vi "Auto-Fill.vi"() -> ()   [LabVIEW 2011]
uses:
  SubVI/Auto-Fill Cases.ctl
  SubVI/Valve_Pump.ctl
  SubVI/Pumps_Valves_Dependencies_Global.vi
panel:
  out "Output Height cm":dbl
  out "Litre":dbl
  in  "Emergency Stop":bool
  out "Litres":dbl(slide) scale=0.0..14400.0
  out "Tank C":dbl(slide) scale=0.0..100.0
  out "Tank B":dbl(slide) scale=0.0..100.0
  out "Tank D":dbl(slide) scale=0.0..100.0
  out "Tank A":dbl(slide) scale=0.0..100.0
  in  "Density (kg/m3)":dbl[](array[numeric])=[0.0, 0.0, 0.0, 0.0, 0.0, 0.0]
  in  "Height (cm)":dbl[](array[numeric])=[0.0, 0.0, 0.0, 0.0, 0.0, 0.0]
  in  "Auto-Fill":T1
  in  "Start Process":bool
  # "Enter density required in \nascending order"
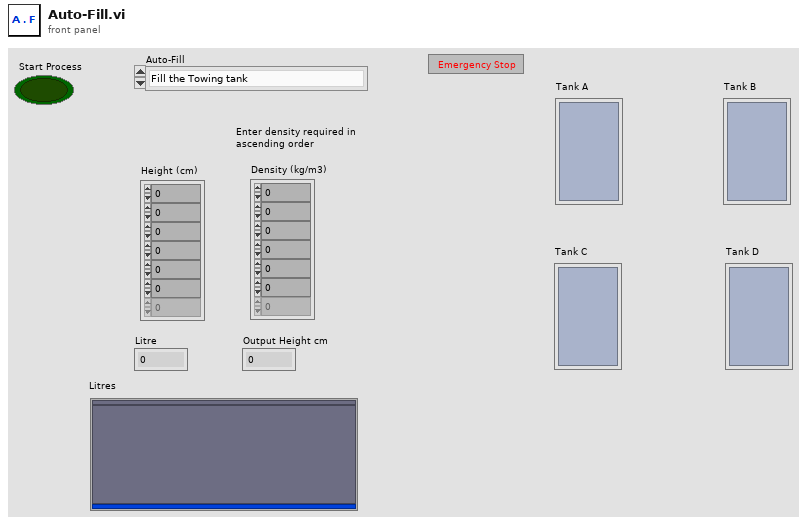
[diagram p1: front panel]
types:
  T1 = typedef "Auto-Fill Cases.ctl" = enum16{"Fill the Towing tank", "Fill Tank A from the Salt saturator tank", "Fill Tank B from the Salt Saturator tank", "Fill Tank C from the water mains", "Fill Tank D from the water mains", "Fill tank B from tank A", "Fill tank C from tank D"}
  T2 = typedef "Valve_Pump.ctl" = enum16{"Main Rack Power", "Pump Power", "Valve Power", "V4", "V5", "V6", "V7", "V8", "V9", "V10", "V11", "V12", "V13", "V14", "V15", "V18", "V19", "V20", "V21", "V22", "V23", "V24", "V25", "V26", "V27", "V28", "V29", "V30", "V31", "V32", "V33", "V34", "Pump A", "Pump B", "Pump C", "Pump D"}
  T3 = cluster{"Tanks[0]":dbl, "Tanks[1]":dbl, "Tanks[2]":dbl, "Tanks[3]":dbl, "Tanks[4]":dbl}
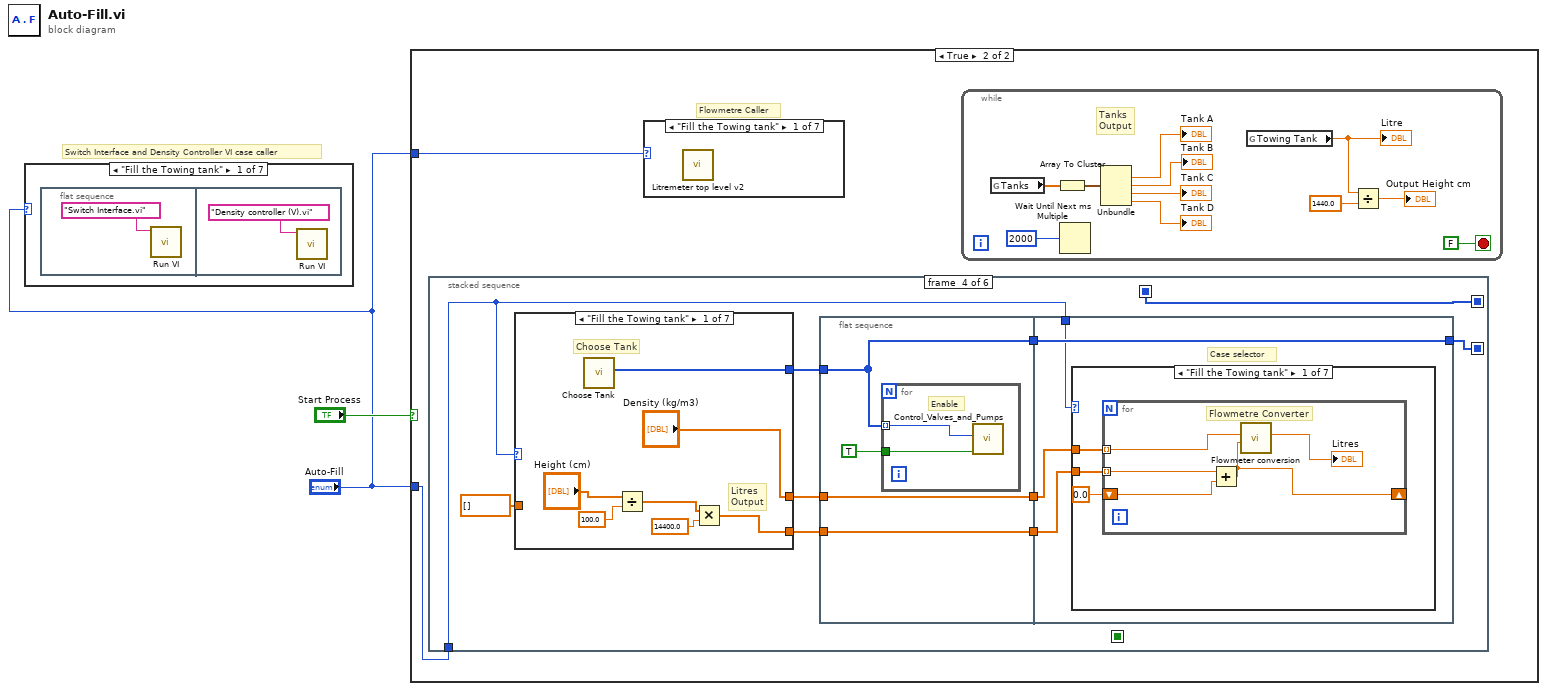
[diagram p0: block diagram]
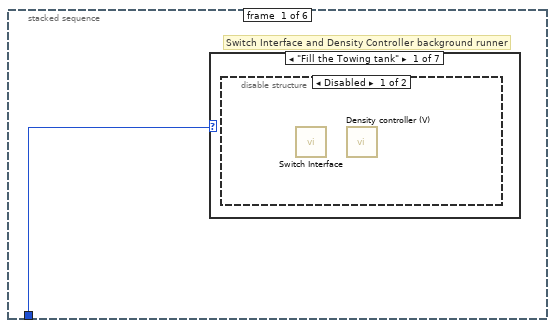
[diagram p15: hidden frame]
diagram:
  # "Switch Interface and Density Controller VI case caller"
  n1 = case shown="\"Fill the Towing tank\"" "Auto-Fill" {
    frame "Fill the Towing tank" {
      n2 = flat-sequence {
        frame #0 {
          n3 = call "Run VI.vi"("VI name"="Switch Interface.vi") -> ()  [unwired: 11 in]
        }
        frame #1 {
          n4 = call "Run VI.vi"("VI name"="Density controller (V).vi") -> ()  [unwired: 11 in]
        }
      }
    }
    frame "Fill Tank A from the Salt saturator tank" {
    }
    frame "Fill Tank B from the Salt Saturator tank" {
    }
    frame "Fill Tank C from the water mains" {
    }
    frame "Fill Tank D from the water mains" {
    }
    frame "Fill tank B from tank A" {
    }
    frame "Fill tank C from tank D" {
    }
  }
  n5 = case shown="True" "Start Process" {
    tunnel: "Auto-Fill" -> [_ w6]
    tunnel: "Auto-Fill" -> [_ w5]
    frame False {
    }
    frame True {
      # "Flowmetre Caller"
      n6 = stacked-sequence {
        seq-local: [_ _ w24 _ _ _] -> [_ _ _ w37 _ _]
        seq-local: [_ _ _ w34 _ _] -> [_ _ _ _ w144 _]
        seq-local: [_ _ _ w37 _ _] -> [_ _ _ _ w143 _]
        seq-local: [_ _ _ _ w140 _] -> [_ _ _ _ _ w148]
        tunnel: w6 -> [w18 _ _ w28 _ _]
        frame #0 {
          # "Switch Interface and Density Controller background runner"
          n7 = case shown="\"Fill the Towing tank\"" w18 {
            frame "Fill the Towing tank" {
              n8 = disable-structure shown="Disabled" {
                frame Disabled {
                  n9 = call "Switch Interface.vi"() -> ()  [unwired: 12 in]
                  n10 = call "Density controller (V).vi"() -> ()  [unwired: 12 in]
                }
                frame Enabled {
                }
              }
            }
            frame "Fill Tank A from the Salt saturator tank" {
            }
            frame "Fill Tank B from the Salt Saturator tank" {
            }
            frame "Fill Tank C from the water mains" {
            }
            frame "Fill Tank D from the water mains" {
            }
            frame "Fill tank B from tank A" {
            }
            frame "Fill tank C from tank D" {
            }
          }
        }
        frame #1 {
          # "Sequence delay time to allow Switch Interface VI to initialize"
          n11 = Wait (ms)(milliseconds to wait=u32 50000 ("millisecond multiple")) -> ()  [unwired: 1 out]
        }
        frame #2 {
          # "Identifier array\nbuild-up"
          n12 = Build Array(Valve_Pump."Main Rack Power" ("Device"), Valve_Pump."Pump Power" ("Device"), Valve_Pump."Valve Power" ("Device")) -> (w24:T2[])
          n13 = for {
            tunnel: TRUE -> [w26]
            tunnel: w24 -> [w27] mode=indexing
            # "Time delay"
            n14 = call "Control_Valves_and_Pumps.vi"("Set state:"=w26, "Device"=w27) -> ()  [unwired: 10 in]
            n15 = Wait Until Next ms Multiple(millisecond multiple=3000) -> ()  [unwired: 1 out]
          }
        }
        frame #3 {
          n16 = case shown="\"Fill the Towing tank\"" w28 {
            tunnel: [w110 w112 w117 w122 w125 w129 w135] -> w35
            tunnel: [w104 w111 w116 w121 w124 w127 w133] -> w29
            tunnel: ["Density (kg/m3)" w111 w116 w121 w124 w127 w133] -> w32
            tunnel: dbl[] [] ("Density (kg/m3)") -> [_ w111 w116 w121 w124 w127 w133]
            frame "Fill the Towing tank" {
              # "Choose Tank"
              # "Litres\nOutput"
              n17 = call "Choose Tank.vi"() -> ("Device"=w110:T2[])  [unwired: 9 in]
              n18 = Divide(x="Height (cm)", y=100.0) -> (x/y=w106:dbl[])
              n19 = Multiply(x=w106, y=14400.0) -> (x*y=w104:dbl[])
            }
            frame "Fill Tank A from the Salt saturator tank" {
              n20 = Build Array(Valve_Pump."V29" ("Device"), Valve_Pump."V27" ("Device"), Valve_Pump."Pump A" ("Device")) -> (w112:T2[])
            }
            frame "Fill Tank B from the Salt Saturator tank" {
              n21 = Build Array(Valve_Pump."V29" ("Device"), Valve_Pump."V23" ("Device"), Valve_Pump."Pump A" ("Device")) -> (w117:T2[])
            }
            frame "Fill Tank C from the water mains" {
              # "Identifier array\nbuild-up"
              n22 = Build Array(Valve_Pump."V8" ("Device")) -> (w122:T2[])
            }
            frame "Fill Tank D from the water mains" {
              # "Identifier array\nbuild-up"
              n23 = Build Array(Valve_Pump."V10" ("Device")) -> (w125:T2[])
            }
            frame "Fill tank B from tank A" {
              # "Identifier array\nbuild-up"
              n24 = Build Array(Valve_Pump."V4" ("Device"), Valve_Pump."V20" ("Device"), Valve_Pump."V22" ("Device"), Valve_Pump."Pump B" ("Device")) -> (w129:T2[])
            }
            frame "Fill tank C from tank D" {
              # "Identifier array\nbuild-up"
              n25 = Build Array(Valve_Pump."V9" ("Device"), Valve_Pump."V15" ("Device"), Valve_Pump."V20" ("Device"), Valve_Pump."V24" ("Device"), Valve_Pump."Pump B" ("Device")) -> (w135:T2[])
            }
          }
          n26 = flat-sequence {
            tunnel: [w40] -> w36
            tunnel: w35 -> [w40]
            tunnel: [w39] -> w33
            tunnel: w32 -> [w39]
            tunnel: [w38] -> w31
            tunnel: w29 -> [w38]
            tunnel: w36 -> [w47]
            tunnel: [w47] -> w34
            tunnel: w33 -> [w46]
            tunnel: w31 -> [w45]
            tunnel: w28 -> [w44]
            frame #0 {
              n27 = for {
                tunnel: w40 -> [w43] mode=indexing
                tunnel: TRUE -> [w42]
                # "Enable"
                n28 = call "Control_Valves_and_Pumps.vi"("Set state:"=w42, "Device"=w43) -> ()  [unwired: 10 in]
              }
            }
            frame #1 {
              # "Case selector"
              n29 = case shown="\"Fill the Towing tank\"" w44 {
                tunnel: w46 -> [w50 _ _ _ _ _ _]
                tunnel: w45 -> [w49 _ _ _ _ _ _]
                frame "Fill the Towing tank" {
                  n30 = for {
                    tunnel: w49 -> [w54] mode=indexing
                    tunnel: w50 -> [w55] mode=indexing
                    shift-right: [w53] -> _
                    shift-left: 0.0 -> [w52]
                    # "Flowmetre Converter"
                    n31 = Add(x=w54, y=w52) -> (x+y=w53:dbl)
                    n32 = call "Flowmeter conversion.vi"("Required Litres"=w53, "Density Required"=w55) -> ("Total Litres (calc)"=→"Litres":dbl)  [unwired: 9 in]
                  }
                }
                frame "Fill Tank A from the Salt saturator tank" {
                  n33 = while {
                    stop <- w58 continue-if-true
                    n34 = flat-sequence {
                      tunnel: [w61] -> w59
                      frame #0 {
                        n35 = call "Tank height conversion.vi"() -> ()  [unwired: 11 in, 1 out]
                      }
                      frame #1 {
                        # "Full case checker"
                        n36 = global read "Pumps_Valves_Dependencies_Global.vi" "Tank A"() -> (w63:dbl)
                        n37 = Less?(x=w63, y=90.0) -> (x < y?=w61:bool)
                      }
                    }
                    n38 = Wait Until Next ms Multiple(millisecond multiple=2000) -> ()  [unwired: 1 out]
                    n39 = local read "Emergency Stop"() -> (w56:bool)
                    n40 = Not(x=w56) -> (.not. x?=w57:bool)
                    n41 = And(x=w59, y=w57) -> (x .and. y?=w58:bool)
                  }
                }
                frame "Fill Tank B from the Salt Saturator tank" {
                  n42 = while {
                    stop <- w66 continue-if-true
                    n43 = flat-sequence {
                      tunnel: [w70] -> w67
                      frame #0 {
                        n44 = call "Tank height conversion.vi"() -> ()  [unwired: 11 in, 1 out]
                      }
                      frame #1 {
                        # "Full case checker"
                        n45 = global read "Pumps_Valves_Dependencies_Global.vi" "Tank B"() -> (w69:dbl)
                        n46 = Less?(x=w69, y=80.0) -> (x < y?=w70:bool)
                      }
                    }
                    n47 = Wait Until Next ms Multiple(millisecond multiple=2000) -> ()  [unwired: 1 out]
                    n48 = local read "Emergency Stop"() -> (w64:bool)
                    n49 = Not(x=w64) -> (.not. x?=w65:bool)
                    n50 = And(x=w67, y=w65) -> (x .and. y?=w66:bool)
                  }
                }
                frame "Fill Tank C from the water mains" {
                  n51 = while {
                    stop <- w74 continue-if-true
                    n52 = flat-sequence {
                      tunnel: [w77] -> w75
                      frame #0 {
                        n53 = call "Tank height conversion.vi"() -> ()  [unwired: 11 in, 1 out]
                      }
                      frame #1 {
                        # "Full case checker"
                        n54 = global read "Pumps_Valves_Dependencies_Global.vi" "Tank C"() -> (w79:dbl)
                        n55 = Less?(x=w79, y=90.0) -> (x < y?=w77:bool)
                      }
                    }
                    n56 = Wait Until Next ms Multiple(millisecond multiple=2000) -> ()  [unwired: 1 out]
                    n57 = Not(x="Emergency Stop") -> (.not. x?=w73:bool)
                    n58 = And(x=w75, y=w73) -> (x .and. y?=w74:bool)
                  }
                }
                frame "Fill Tank D from the water mains" {
                  n59 = while {
                    stop <- w82 continue-if-true
                    n60 = flat-sequence {
                      tunnel: [w85] -> w83
                      frame #0 {
                        n61 = call "Tank height conversion.vi"() -> ()  [unwired: 11 in, 1 out]
                      }
                      frame #1 {
                        # "Full case checker"
                        n62 = global read "Pumps_Valves_Dependencies_Global.vi" "Tank D"() -> (w87:dbl)
                        n63 = Less?(x=w87, y=90.0) -> (x < y?=w85:bool)
                      }
                    }
                    n64 = Wait Until Next ms Multiple(millisecond multiple=2000) -> ()  [unwired: 1 out]
                    n65 = local read "Emergency Stop"() -> (w80:bool)
                    n66 = Not(x=w80) -> (.not. x?=w81:bool)
                    n67 = And(x=w83, y=w81) -> (x .and. y?=w82:bool)
                  }
                }
                frame "Fill tank B from tank A" {
                  n68 = while {
                    stop <- w90 continue-if-true
                    n69 = flat-sequence {
                      tunnel: [w93] -> w91
                      frame #0 {
                        n70 = call "Tank height conversion.vi"() -> ()  [unwired: 11 in, 1 out]
                      }
                      frame #1 {
                        # "Full case checker"
                        n71 = global read "Pumps_Valves_Dependencies_Global.vi" "Tank B"() -> (w95:dbl)
                        n72 = Less?(x=w95, y=90.0) -> (x < y?=w93:bool)
                      }
                    }
                    n73 = Wait Until Next ms Multiple(millisecond multiple=2000) -> ()  [unwired: 1 out]
                    n74 = local read "Emergency Stop"() -> (w88:bool)
                    n75 = Not(x=w88) -> (.not. x?=w89:bool)
                    n76 = And(x=w91, y=w89) -> (x .and. y?=w90:bool)
                  }
                }
                frame "Fill tank C from tank D" {
                  n77 = while {
                    stop <- w98 continue-if-true
                    n78 = flat-sequence {
                      tunnel: [w101] -> w99
                      frame #0 {
                        n79 = call "Tank height conversion.vi"() -> ()  [unwired: 11 in, 1 out]
                      }
                      frame #1 {
                        # "Full case checker"
                        n80 = global read "Pumps_Valves_Dependencies_Global.vi" "Tank C"() -> (w103:dbl)
                        n81 = Less?(x=w103, y=90.0) -> (x < y?=w101:bool)
                      }
                    }
                    n82 = Wait Until Next ms Multiple(millisecond multiple=2000) -> ()  [unwired: 1 out]
                    n83 = local read "Emergency Stop"() -> (w97:bool)
                    n84 = Not(x=w97) -> (.not. x?=w96:bool)
                    n85 = And(x=w99, y=w96) -> (x .and. y?=w98:bool)
                  }
                }
              }
            }
          }
        }
        frame #4 {
          w140 = FALSE ("Set state:")
          # "Identifier array inverse\nbuild-up"
          n86 = Build Array (concatenate)(w143, w144) -> (w142:T2[])
          n87 = Reverse 1D Array(array=w142) -> (reversed array=w141:T2[])
          n88 = for {
            tunnel: w140 -> [w147]
            tunnel: w141 -> [w146] mode=indexing
            # "Time delay"
            n89 = call "Control_Valves_and_Pumps.vi"("Set state:"=w147, "Device"=w146) -> ()  [unwired: 10 in]
            n90 = Wait Until Next ms Multiple(millisecond multiple=5000) -> ()  [unwired: 1 out]
          }
        }
        frame #5 {
          n91 = local write "Start Process"(w148) -> ()
        }
      }
      n92 = case shown="\"Fill the Towing tank\"" w5 {
        frame "Fill the Towing tank" {
          n93 = call "Litremeter top level v2.vi"() -> ()  [unwired: 1 in]
        }
        frame "Fill Tank A from the Salt saturator tank" {
        }
        frame "Fill Tank B from the Salt Saturator tank" {
        }
        frame "Fill Tank C from the water mains" {
        }
        frame "Fill Tank D from the water mains" {
        }
        frame "Fill tank B from tank A" {
        }
        frame "Fill tank C from tank D" {
        }
      }
      n94 = while {
        stop <- FALSE stop-if-true
        # "Tanks \nOutput"
        n95 = global read "Pumps_Valves_Dependencies_Global.vi" "Tanks"() -> (w16:dbl[])
        n96 = Array To Cluster(array=w16) -> (cluster=w17:T3)
        n97 = Wait Until Next ms Multiple(millisecond multiple=2000) -> ()  [unwired: 1 out]
        n98 = Unbundle(w17) -> ("Tanks[1]"=→"Tank A":dbl, "Tanks[2]"=→"Tank B":dbl, "Tanks[3]"=→"Tank C":dbl, "Tanks[4]"=→"Tank D":dbl)  [unwired: 1 out]
        n99 = global read "Pumps_Valves_Dependencies_Global.vi" "Towing Tank"() -> (w8:dbl)
        "Litre" <- w8
        n100 = Divide(x=w8, y=1440.0) -> (x/y=→"Output Height cm":dbl)
      }
    }
  }
